vi "Write Simple Address.vi"(8 "error in (no error)":errorcluster, 10 "Simple Address":i32, 11 "Enumeration Tree Queue Mailman in":refnum<class "Enumeration Tree Queue Mailman.lvclass">) -> (0 "error out":errorcluster, 3 "Enumeration Tree Queue Mailman out":refnum<class "Enumeration Tree Queue Mailman.lvclass">)   [LabVIEW 2024, in "Enumeration Tree Queue Mailman.lvclass"]
uses:
  Enumeration Tree Queue Mailman.lvclass
  Simple Tree Queue Mailman/Simple Tree Queue Mailman.lvclass
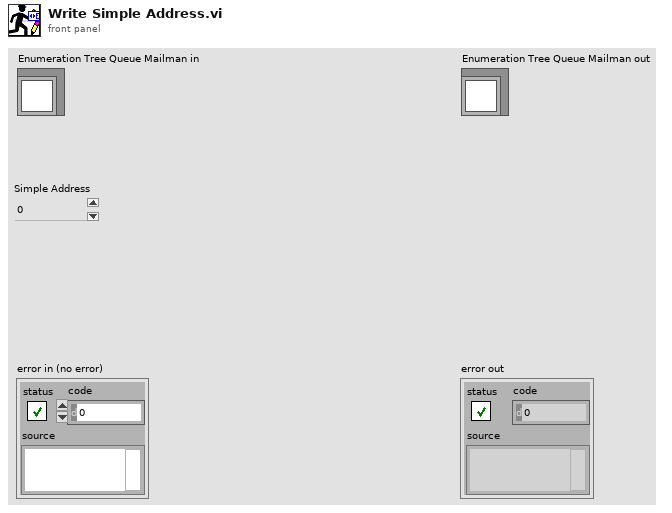
[diagram p1: front panel]
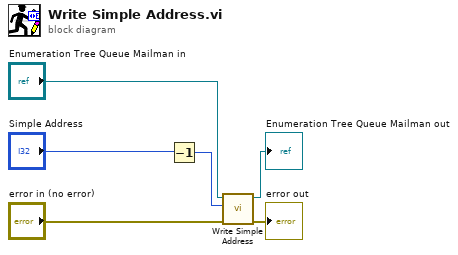
[diagram p0: block diagram]
diagram:
  n1 = Decrement(x="Simple Address") -> (x-1=w2:i32)
  n2 = call-parent "Write Simple Address.vi"("error in (no error)"="error in (no error)", "Simple Address"=w2, "Simple Tree Queue Mailman in"="Enumeration Tree Queue Mailman in") -> ("error out"=→"error out":errorcluster, "Simple Tree Queue Mailman out"=→"Enumeration Tree Queue Mailman out":refnum<class "Enumeration Tree Queue Mailman.lvclass">)  [unwired: 7 in]
